vi "Send_AC.vi"(5 "milliseconds to wait":u32=5000, 8 "error in (no error)":errorcluster, 11 "DataSocketCluster In":T1={"Server Machine"="siskin", "Client Machine"="becard", "Data"="P2", "TimeStamp"=0.0, "Count"=0, "Target Process"="General Server"} {"TimeStamp" format="%.2f"}) -> (0 "error out":errorcluster {"code" format="%.0x"}, 1 "Response to SEND AC":string, 3 "DataSocketCluster out":T1={"Server Machine"="siskin", "Client Machine"="becard", "Data"="P2", "TimeStamp"=0.0, "Count"=0, "Target Process"="General Server"} {"TimeStamp" format="%.2f"})   [LabVIEW 2020]
uses:
  DataSocketCluster external.ctl
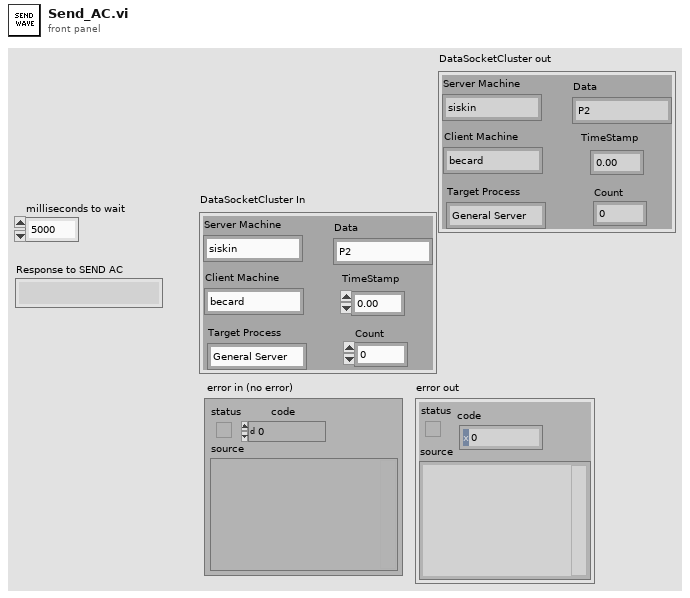
[diagram p1: front panel]
types:
  T1 = typedef "DataSocketCluster external.ctl" = cluster{"Server Machine":string, "Client Machine":string, "Data":string, "TimeStamp":dbl, "Count":i32, "Target Process":string}
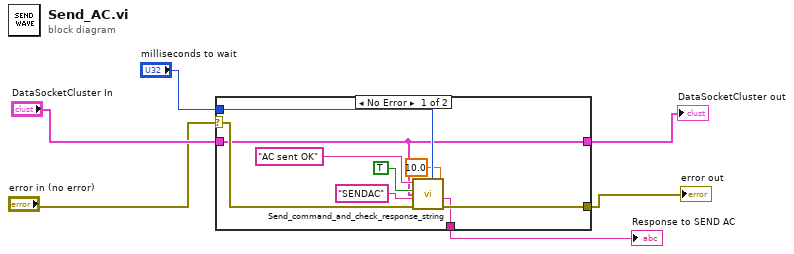
[diagram p0: block diagram]
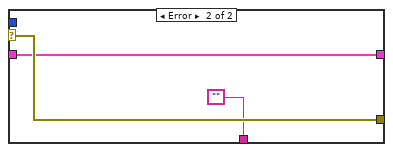
[diagram p2: hidden frame]
diagram:
  n1 = case shown="No Error" "error in (no error)" {
    selector: "error in (no error)" -> [w11 w18]
    tunnel: [w12 w18] -> w6
    tunnel: "DataSocketCluster In" -> [w8 w16]
    tunnel: "milliseconds to wait" -> [w10 _]
    tunnel: [w9 ""] -> w2
    tunnel: [w8 w16] -> w1
    frame No Error {
      n2 = call "Send_command_and_check_response_string.vi"("TimeOut Time (s)"=10.0, "milliseconds to wait"=w10, "output cluster"=w8, "error in (no error)"=w11, "Command"="SENDAC", "test response?"=TRUE, "Expected response"="AC sent OK" ("x")) -> ("error IO"=w12:errorcluster, "Return value"=w9:string)  [unwired: 1 in]
    }
    frame Error {
    }
  }
  "error out" <- w6
  "Response to SEND AC" <- w2
  "DataSocketCluster out" <- w1
